vi "programa10.vi"() -> ()   [LabVIEW 2011]
uses:
  <vilib>/express/express arith-compare/Formula/XNode/ExpressFormulaBlockNode.xnode
panel:
  out "Contador":dbl
  out "Par":bool
  out "Impar":bool
  out "Contador Impares":dbl
  out "Contador Pares":dbl
  out "Numero":dbl
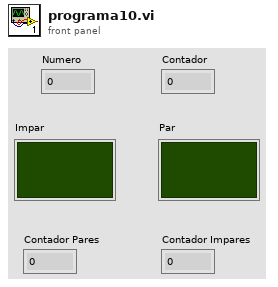
[diagram p1: front panel]
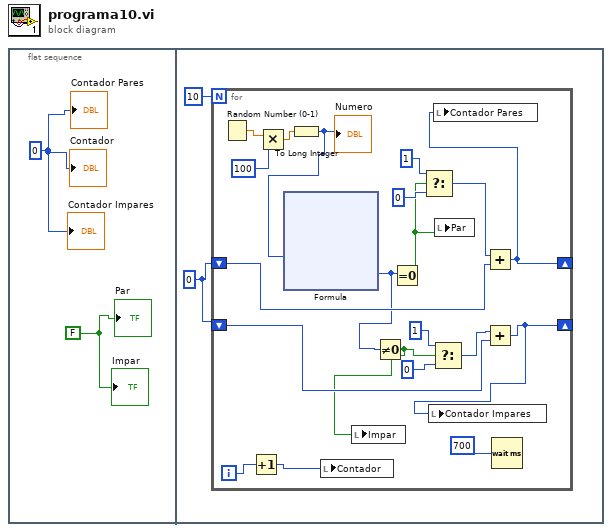
[diagram p0: block diagram]
diagram:
  n1 = flat-sequence {
    frame #0 {
      w1 = FALSE
      w2 = 0
      "Impar" <- w1
      "Par" <- w1
      "Contador Pares" <- w2
      "Contador" <- w2
      "Contador Impares" <- w2
    }
    frame #1 {
      w3 = 0
      n2 = for {
        N: 10 -> [_]
        shift-right: [w16] -> _
        shift-left: w3 -> [w17]
        shift-right: [w10] -> _
        shift-left: w3 -> [w11]
        i -> [w6]
        n3 = Random Number (0-1)() -> (number: 0 to 1=w23:dbl)
        n4 = Increment(x=w6) -> (x+1=w5:i32)
        n5 = Multiply(x=w23, y=100) -> (x*y=w22:dbl)
        n6 = To Long Integer(number=w22) -> (32bit integer=w21:i32)
        "Numero" <- w21
        n7 = xnode "Formula"("X1"=w21) -> ("Result"=w13:i32)  [unwired: 1 in, 1 out]
        n8 = local write "Contador"(w5) -> ()
        n9 = Not Equal To 0?(x=w13) -> (x != 0?=w9:bool)
        n10 = local write "Impar"(w9) -> ()
        n11 = Equal To 0?(x=w13) -> (x = 0?=w8:bool)
        n12 = Select(t=1, s=w8, f=0) -> (s? t:f=w18:i32)
        n13 = Select(t=1, s=w9, f=0) -> (s? t:f=w12:i32)
        n14 = local write "Par"(w8) -> ()
        n15 = Add(x=w18, y=w17) -> (x+y=w16:i32)
        n16 = local write "Contador Pares"(w16) -> ()
        n17 = Add(x=w12, y=w11) -> (x+y=w10:i32)
        n18 = local write "Contador Impares"(w10) -> ()
        n19 = Wait (ms)(milliseconds to wait=700) -> ()  [unwired: 1 out]
      }
    }
  }
